vi "get_FTPSettings.vi"(0 "Host_Reference":refnum<class "HGF_Reference.lvclass">, 2 "timeout in ms (-1)":i32=-1, 5 "error in (no error)":errorcluster) -> (14 "dup Host_Reference":refnum<class "HGF_Reference.lvclass">, 16 "FTP Settings":T1, 19 "error out":errorcluster)   [LabVIEW 2009, in "MoAgSy.lvlib" / "MoAgSy_Host.lvclass"]
doc: "<B>public</B> VI returns FTP settings from referenced Host.\nFTP settings are needed to download unknown class code dynamically.\n\nF.Berck@gsi.de\nGSI Darmstadt 2009"
uses:
  MoAgSy_Host.lvclass
  HGF_BaseClasses/HGF_Reference/HGF_Reference.lvclass
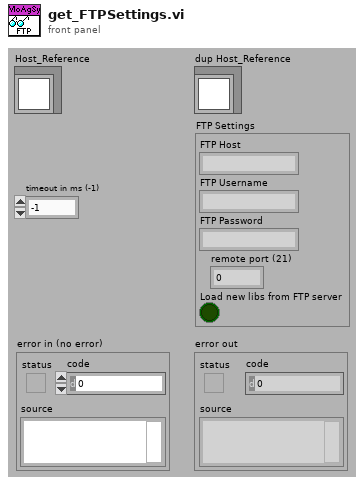
[diagram p1: front panel]
types:
  T1 = cluster{"FTP Host":string, "FTP Username":string, "FTP Password":string, "remote port (21)":u16, "Load new libs from FTP server":bool}
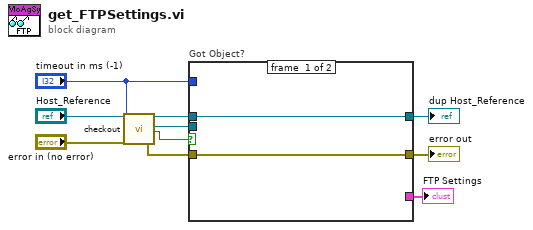
[diagram p0: block diagram]
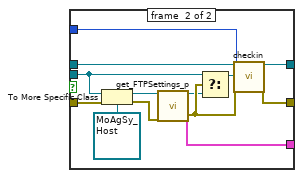
[diagram p2: hidden frame]
diagram:
  n1 = call "checkout.vi"("HGF_Reference"="Host_Reference", "timeout in ms (-1)"="timeout in ms (-1)", "error in (no error)"="error in (no error)") -> ("dup HGF_Reference"=w5:refnum<class "HGF_Reference.lvclass">, "Object"=w8:refnum<class>, "got object?"=w6:bool, "error out"=w9:errorcluster)  [unwired: 13 out]
  n2 = case "Got Object?" shown="True" w6 {
    tunnel: w9 -> [w11 w24]
    tunnel: w8 -> [_ w14]
    tunnel: [_ w16] -> w1
    tunnel: w5 -> [w12 w20]
    tunnel: [w12 w19] -> w4
    tunnel: "timeout in ms (-1)" -> [_ w18]
    tunnel: [w11 w17] -> w2
    frame #0 {
    }
    frame #1 {
      n3 = To More Specific Class(target class=refnum<class "MoAgSy_Host.lvclass"> refnum ("MoAgSy.lvlib:MoAgSy_Host.lvclass"), reference=w14, error in=w24) -> (specific class reference=w22:refnum<class "MoAgSy_Host.lvclass">, error out=w21:errorcluster)
      n4 = call "get_FTPSettings_p.vi"("MoAgSy_Host"=w22, "error in (no error)"=w21) -> ("dup MoAgSy_Host"=w15:refnum<class "MoAgSy_Host.lvclass">, "FTP Settings"=w16:T1, "error out"=w25:errorcluster)  [unwired: 15 out]
      n5 = Select(t=w14, s=w25, f=w15) -> (s? t:f=w13:refnum<class>)
      n6 = call "checkin.vi"("HGF_Reference"=w20, "Object"=w13, "timeout /ms (-1)"=w18, "error in (no error)"=w25) -> ("dup HGF_Reference"=w19:refnum<class "HGF_Reference.lvclass">, "error out"=w17:errorcluster)  [unwired: 14 out]
    }
  }
  "dup Host_Reference" <- w4
  "error out" <- w2
  "FTP Settings" <- w1
